vi "LH_InsertBackIndex.vi"(1 "Index":i32, 2 "InsertContent":i32, 3 "InputList":refnum<class "ListHead.lvclass">) -> (0 "OutputList":refnum<class "ListHead.lvclass">)   [LabVIEW 2014, in "ListHead.lvclass"]
uses:
  ListHead.lvclass
  ListHead.lvclass/ListHead.ctl
  ListNode.lvclass
  ListNodeVirtual.lvclass
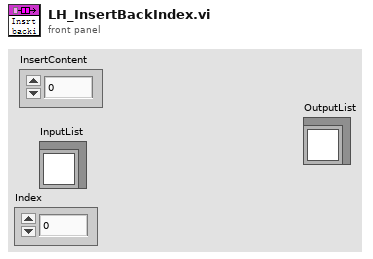
[diagram p1: front panel]
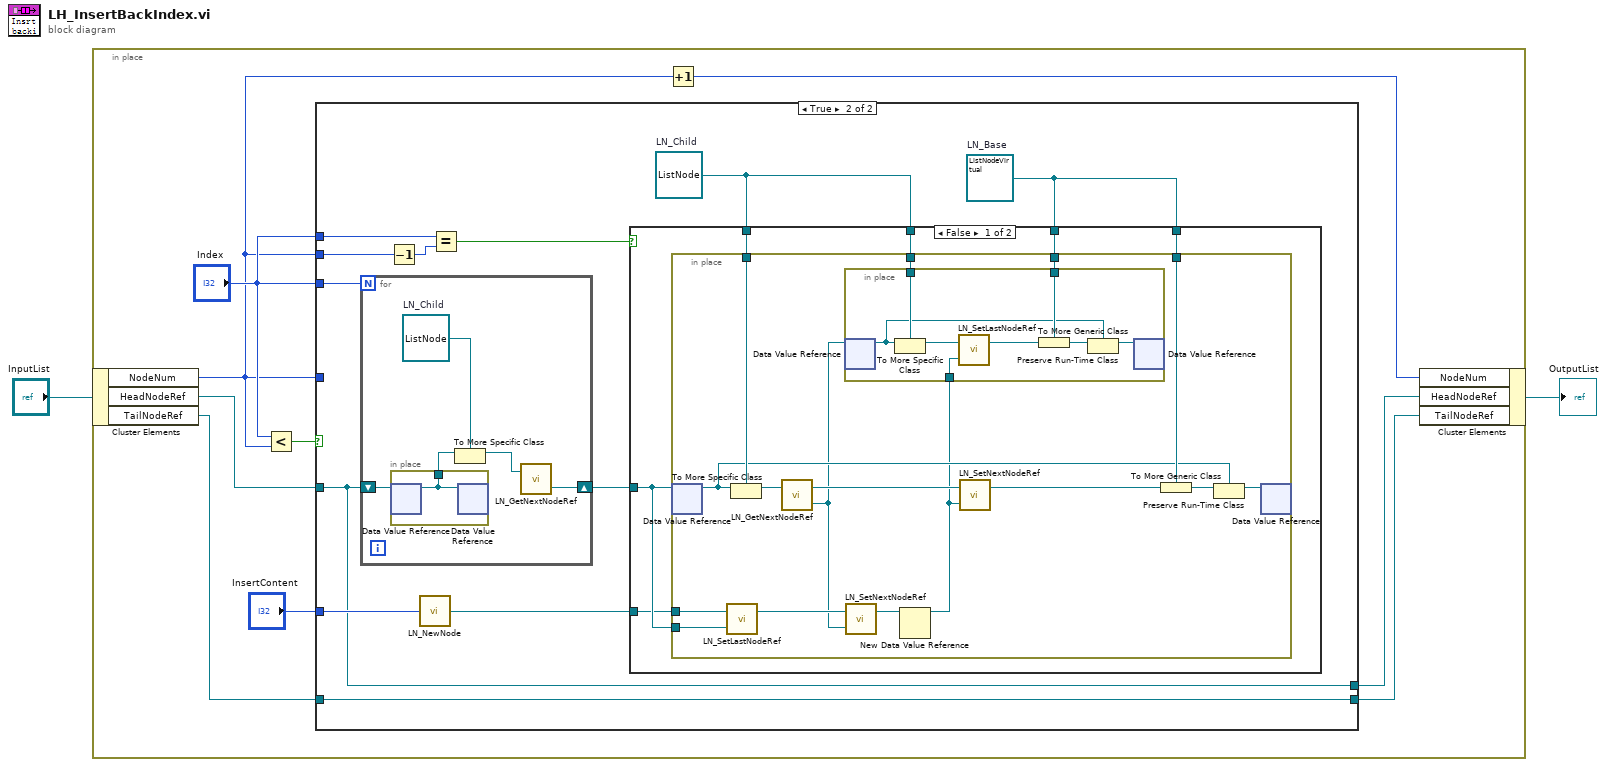
[diagram p0: block diagram]
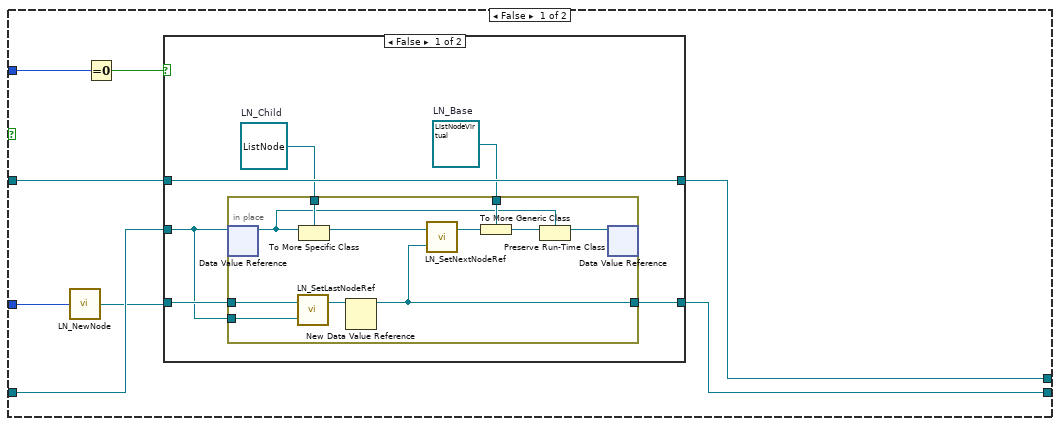
[diagram p2: hidden frame]
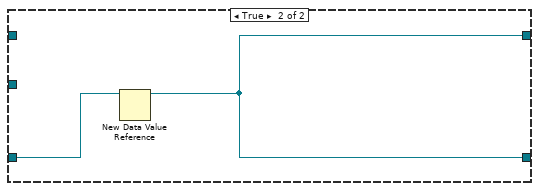
[diagram p3: hidden frame]
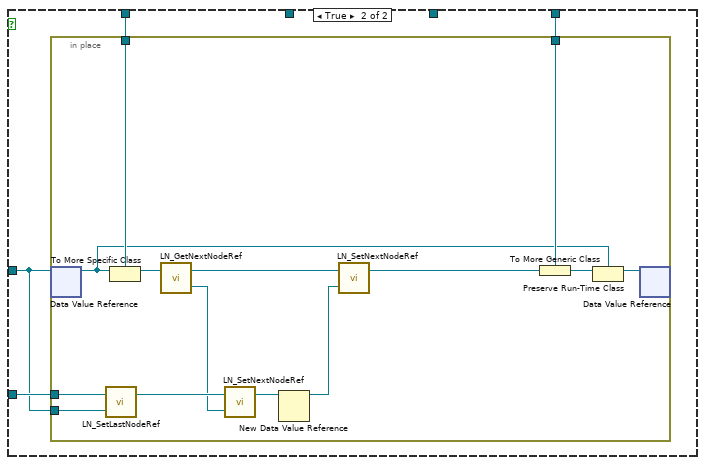
[diagram p4: hidden frame]
diagram:
  n1 = in-place {
    n2 = in-place-cluster #1("InputList") -> ("NodeNum"=w3:u32, "HeadNodeRef"=w9:refnum<data-value>, "TailNodeRef"=w8:refnum<data-value>)
    n3 = Less?(x="Index", y=w3) -> (x < y?=w10:bool)
    n4 = case shown="True" w10 {
      tunnel: w9 -> [w17 w47]
      tunnel: "Index" -> [_ w45]
      tunnel: "InsertContent" -> [w15 w50]
      tunnel: w8 -> [w16 w46]
      tunnel: [w13 w47] -> w6
      tunnel: [w12 w46] -> w5
      tunnel: w3 -> [w19 _]
      tunnel: "Index" -> [_ w44]
      tunnel: w3 -> [_ w42]
      frame False {
        n5 = call "LN_NewNode.vi"("InputContent"=w15) -> ("OutputListNode"=w14:refnum<class "ListNode.lvclass">)
        n6 = Equal To 0?(x=w19) -> (x = 0?=w18:bool)
        n7 = case shown="False" w18 {
          tunnel: w14 -> [w22 w38]
          tunnel: w17 -> [w25 _]
          tunnel: w16 -> [w21 _]
          tunnel: [w24 w37] -> w12
          tunnel: [w25 w37] -> w13
          frame False {
            w20 = refnum<class "ListNodeVirtual.lvclass"> refnum  # LN_Base
            w23 = refnum<class "ListNode.lvclass"> refnum  # LN_Child
            n8 = in-place {
              in-place-border: [w31] -> w24
              in-place-border: w23 -> [w36]
              in-place-border: w22 -> [w34]
              in-place-border: w21 -> [w33]
              in-place-border: w20 -> [w30]
              n9 = in-place-dvr #2(w21) -> (w27:refnum<class "ListNodeVirtual.lvclass">)  [unwired: 1 out]
              n10 = call "LN_SetLastNodeRef.vi"("InputLastNodeRef"=w33, "InputListNode"=w34) -> ("OutputListNode"=w32:refnum<class "ListNode.lvclass">)  [unwired: 1 in]
              n11 = To More Specific Class(target class=w36, reference=w27) -> (specific class reference=w35:refnum<class "ListNode.lvclass">)  [unwired: 1 in, 1 out]
              n12 = New Data Value Reference(data value=w32) -> (data value reference=w31:refnum<data-value>)  [unwired: 1 in, 1 out]
              n13 = call "LN_SetNextNodeRef.vi"("InputNextNodeRef"=w31, "InputListNode"=w35) -> ("OutputListNode"=w29:refnum<class "ListNode.lvclass">)  [unwired: 1 in]
              n14 = To More Generic Class(target class=w30, reference=w29) -> (generic class reference=w28:refnum<class "ListNodeVirtual.lvclass">)
              n15 = Preserve Run-Time Class(object in=w28, 2:w27) -> (object out=w26:refnum<class "ListNodeVirtual.lvclass">)  [unwired: 1 in, 1 out]
              n16 = in-place-dvr #2(w26) -> ()  [unwired: 2 out]
            }
          }
          frame True {
            n17 = New Data Value Reference(data value=w38) -> (data value reference=w37:refnum<data-value>)  [unwired: 1 in, 1 out]
          }
        }
      }
      frame True {
        w39 = refnum<class "ListNodeVirtual.lvclass"> refnum  # LN_Base
        w40 = refnum<class "ListNode.lvclass"> refnum  # LN_Child
        n18 = for {
          N: w45 -> [_]
          shift-right: [w99] -> w48
          shift-left: w47 -> [w103]
          w102 = refnum<class "ListNode.lvclass"> refnum  # LN_Child
          n19 = in-place {
            in-place-border: [w104] -> w101
            n20 = in-place-dvr #3(w103) -> (w104:refnum<class "ListNodeVirtual.lvclass">)  [unwired: 1 out]
            n21 = in-place-dvr #3(w104) -> ()  [unwired: 2 out]
          }
          n22 = To More Specific Class(target class=w102, reference=w101) -> (specific class reference=w100:refnum<class "ListNode.lvclass">)  [unwired: 1 in, 1 out]
          n23 = call "LN_GetNextNodeRef.vi"("InputListNode"=w100) -> ("OutputNextNodeRef"=w99:refnum<data-value>)  [unwired: 1 in, 1 out]
        }
        n24 = Decrement(x=w42) -> (x-1=w43:u32)
        n25 = call "LN_NewNode.vi"("InputContent"=w50) -> ("OutputListNode"=w49:refnum<class "ListNode.lvclass">)
        n26 = Equal?(x=w44, y=w43) -> (x = y?=w41:bool)
        n27 = case shown="False" w41 {
          tunnel: w40 -> [w54 w84]
          tunnel: w49 -> [w55 w83]
          tunnel: w48 -> [w56 w82]
          tunnel: w39 -> [w53 w81]
          tunnel: w40 -> [w52 _]
          tunnel: w39 -> [w51 _]
          frame False {
            n28 = in-place {
              in-place-border: w54 -> [w72]
              in-place-border: w55 -> [w70]
              in-place-border: w56 -> [w69]
              in-place-border: w53 -> [w64]
              in-place-border: w52 -> [w59]
              in-place-border: w51 -> [w57]
              n29 = in-place-dvr #4(w56) -> (w62:refnum<class "ListNodeVirtual.lvclass">)  [unwired: 1 out]
              n30 = call "LN_SetLastNodeRef.vi"("InputLastNodeRef"=w69, "InputListNode"=w70) -> ("OutputListNode"=w68:refnum<class "ListNode.lvclass">)  [unwired: 1 in]
              n31 = To More Specific Class(target class=w72, reference=w62) -> (specific class reference=w71:refnum<class "ListNode.lvclass">)  [unwired: 1 in, 1 out]
              n32 = call "LN_GetNextNodeRef.vi"("InputListNode"=w71) -> ("OutputNextNodeRef"=w60:refnum<data-value>, "OutputListNode"=w66:refnum<class "ListNode.lvclass">)  [unwired: 1 in]
              n33 = call "LN_SetNextNodeRef.vi"("InputNextNodeRef"=w60, "InputListNode"=w68) -> ("OutputListNode"=w67:refnum<class "ListNode.lvclass">)  [unwired: 1 in]
              n34 = New Data Value Reference(data value=w67) -> (data value reference=w58:refnum<data-value>)  [unwired: 1 in, 1 out]
              n35 = in-place {
                in-place-border: w59 -> [w80]
                in-place-border: w58 -> [w78]
                in-place-border: w57 -> [w76]
                n36 = in-place-dvr #5(w60) -> (w73:refnum<class "ListNodeVirtual.lvclass">)  [unwired: 1 out]
                n37 = To More Specific Class(target class=w80, reference=w73) -> (specific class reference=w79:refnum<class "ListNode.lvclass">)  [unwired: 1 in, 1 out]
                n38 = call "LN_SetLastNodeRef.vi"("InputLastNodeRef"=w78, "InputListNode"=w79) -> ("OutputListNode"=w77:refnum<class "ListNode.lvclass">)  [unwired: 1 in]
                n39 = To More Generic Class(target class=w76, reference=w77) -> (generic class reference=w75:refnum<class "ListNodeVirtual.lvclass">)
                n40 = Preserve Run-Time Class(object in=w75, 2:w73) -> (object out=w74:refnum<class "ListNodeVirtual.lvclass">)  [unwired: 1 in, 1 out]
                n41 = in-place-dvr #5(w74) -> ()  [unwired: 2 out]
              }
              n42 = call "LN_SetNextNodeRef.vi"("InputNextNodeRef"=w58, "InputListNode"=w66) -> ("OutputListNode"=w65:refnum<class "ListNode.lvclass">)  [unwired: 1 in]
              n43 = To More Generic Class(target class=w64, reference=w65) -> (generic class reference=w63:refnum<class "ListNodeVirtual.lvclass">)
              n44 = Preserve Run-Time Class(object in=w63, 2:w62) -> (object out=w61:refnum<class "ListNodeVirtual.lvclass">)  [unwired: 1 in, 1 out]
              n45 = in-place-dvr #4(w61) -> ()  [unwired: 2 out]
            }
          }
          frame True {
            n46 = in-place {
              in-place-border: w84 -> [w98]
              in-place-border: w83 -> [w96]
              in-place-border: w82 -> [w95]
              in-place-border: w81 -> [w88]
              n47 = in-place-dvr #6(w82) -> (w86:refnum<class "ListNodeVirtual.lvclass">)  [unwired: 1 out]
              n48 = call "LN_SetLastNodeRef.vi"("InputLastNodeRef"=w95, "InputListNode"=w96) -> ("OutputListNode"=w94:refnum<class "ListNode.lvclass">)  [unwired: 1 in]
              n49 = To More Specific Class(target class=w98, reference=w86) -> (specific class reference=w97:refnum<class "ListNode.lvclass">)  [unwired: 1 in, 1 out]
              n50 = call "LN_GetNextNodeRef.vi"("InputListNode"=w97) -> ("OutputNextNodeRef"=w93:refnum<data-value>, "OutputListNode"=w90:refnum<class "ListNode.lvclass">)  [unwired: 1 in]
              n51 = call "LN_SetNextNodeRef.vi"("InputNextNodeRef"=w93, "InputListNode"=w94) -> ("OutputListNode"=w92:refnum<class "ListNode.lvclass">)  [unwired: 1 in]
              n52 = New Data Value Reference(data value=w92) -> (data value reference=w91:refnum<data-value>)  [unwired: 1 in, 1 out]
              n53 = call "LN_SetNextNodeRef.vi"("InputNextNodeRef"=w91, "InputListNode"=w90) -> ("OutputListNode"=w89:refnum<class "ListNode.lvclass">)  [unwired: 1 in]
              n54 = To More Generic Class(target class=w88, reference=w89) -> (generic class reference=w87:refnum<class "ListNodeVirtual.lvclass">)
              n55 = Preserve Run-Time Class(object in=w87, 2:w86) -> (object out=w85:refnum<class "ListNodeVirtual.lvclass">)  [unwired: 1 in, 1 out]
              n56 = in-place-dvr #6(w85) -> ()  [unwired: 2 out]
            }
          }
        }
      }
    }
    n57 = Increment(x=w3) -> (x+1=w7:u32)
    n58 = in-place-cluster #1("NodeNum"=w7, "HeadNodeRef"=w6, "TailNodeRef"=w5) -> (→"OutputList":refnum<class "ListHead.lvclass">)
  }
